vi "LIA Example Host.vi"() -> ()   [LabVIEW 2017]
uses:
  Program Files (x86)/National Instruments/LabVIEW 2017/examples/Lock-In Amplifier/lib/host/Public/pll settings.ctl
  Program Files (x86)/National Instruments/LabVIEW 2017/examples/Lock-In Amplifier/lib/host/Public/lock-in settings.ctl
  Program Files (x86)/National Instruments/LabVIEW 2017/examples/Lock-In Amplifier/lib/interface/Interface FPGA/LIA Host Interface FPGA.lvclass
  C:/Program Files (x86)/National Instruments/LabVIEW 2017/examples/Lock-In Amplifier/lib/interface/Interface/LIA Host Interface.lvclass
  Program Files (x86)/National Instruments/LabVIEW 2017/examples/Lock-In Amplifier/lib/host/Public/fpga type.ctl
  <vilib>/Analysis/4window.llb/windowTd.ctl
  <vilib>/measure/maspectr.llb/Power Spectrum and PSD Export Mode.ctl
  Program Files (x86)/National Instruments/LabVIEW 2017/examples/Lock-In Amplifier/lib/interface/Interface FPGA/Properties/FpgaSession_GET.vi
  <vilib>/Utility/error.llb/Error Cluster From Error Code.vi
  <vilib>/rvi/errors/niLvFpgaAdjustHostInterfaceError.vi
  <vilib>/measure/maspectr.llb/FFT Power Spectrum and PSD for 1 Chan (CDB).vi
  <vilib>/rvi/interface/nirviReadWriteControl/nirviReadWriteControl.xnode
  Program Files (x86)/National Instruments/LabVIEW 2017/examples/Lock-In Amplifier/lib/interface/Interface/LIA Host Interface.lvclass
  Program Files (x86)/National Instruments/LabVIEW 2017/examples/Lock-In Amplifier/lib/host/Lock-In Amplifier Example Host.lvlib
  Program Files (x86)/National Instruments/LabVIEW 2017/examples/Lock-In Amplifier/lib/shared/Lock-In Amplifier Example Shared.lvlib
  NiFpgaLv.dll
  <vilib>/rvi/interface/Simulation/niFpgaSimulationCallBeginRW.vi
  <vilib>/Analysis/NI_AALPro.lvlib
  <vilib>/measure/NI_MAPro.lvlib
  <vilib>/ptbypt/NI_PtbyPt.lvlib
panel:
  in  "Tab Control 2":enum32{"Page 1"}(tab)
  in  "dpll.m 0":i8=-20
  in  "lock-in.decimator 0":enum16{"CIC", "FIR", "None"}(ring)=enum."FIR"
  in  "averaging parameters":T1={"averaging mode"=enum."No averaging", "weighting mode"=enum."Exponential", "number of averages"=10}
  in  "restart averaging (F)":bool
  out "lock-in.max-min":dbl=1.9775797561733533e-07 caption="Deviation" format="%#_6p"
  out "lock-in.min":dbl=1.9775797561733533e-07 caption="Deviation" format="%#_6p"
  out "lock-in.max":dbl=1.9775797561733533e-07 caption="Deviation" format="%#_6p"
  in  "Tab Control 1":enum32{"Page 1", "Page 2"}(tab)
  out "max value":dbl
  out "Waveform Graph 2":cluster{"f0":dbl, "df":dbl, "magnitude":dbl[]}(graph)
  out "stream.request state 0":T2(ring)
  out "pll.vco output 0":fxp<+/-,48,0> format="%#.18g"
  out "lock-in.cic config 0":cluster{"factor":fxp<+,16,16>, "shift":i16}
  out "stream.num samples 0":u64
  out "stream.state 0":T2(ring)
  out "unscaled data":i64[][](array[numeric])
  out "dpll.vco output 0":fxp<+/-,48,0> format="%#.18g"
  out "dpll.config 0":T3
  out "Waveform Graph":cluster{"f0":dbl, "df":dbl, "magnitude":dbl[]}[](graph)
  in  "app.quit":bool
  in  "lock-in.boxcar length 0":u32=2048 caption="Boxar Length"
  in  "app.tab 0":enum32{"Lock-In", "PLL"}(tab)
  in  "lock-in.manual carrier 0":dbl=100000.0 caption="Carrier" format="%_8p"
  in  "lock-in.decimation 0":i32=2048 caption="Decimation"
  in  "lock-in.source 0":enum16{"AI 0", "AI 1", "AI 2", "AI 3"}(ring)=enum."AI 1" caption="Channel"
  in  "lock-in.carrier 0":T4(ring)=enum."DPLL 0" caption="Carrier Source"
  in  "pll.source 0":enum16{"AI 0", "AI 1", "AI 2", "AI 3"}(ring) caption="Source"
  in  "pll.q frequency 0":dbl=100000.0 caption="Q Frequency" format="%#_6p"
  in  "pll.reset 0":bool caption="PLL Reset"
  in  "rio device":tag="PXI1Slot8" caption="Resource"
  in  "lock-in.reset boxar 0":bool
  out "lock-in.deviation 1":dbl=1.9775797561733533e-07 caption="Deviation" format="%#_6p"
  out "lock-in.amplitude 0":dbl=8.221341747482856e-05 caption="Result" format="%#_12p"
  in  "lock-in.boxcar lookback 0":i32=1024 caption="Windows to Average"
  out "Result":cluster{"mean":dbl, "trace":dbl}(graph)={"mean"=8.221341747482856e-05, "trace"=8.36741779633565e-05}
  # "NI Lock-In Amplifier Reference Example"
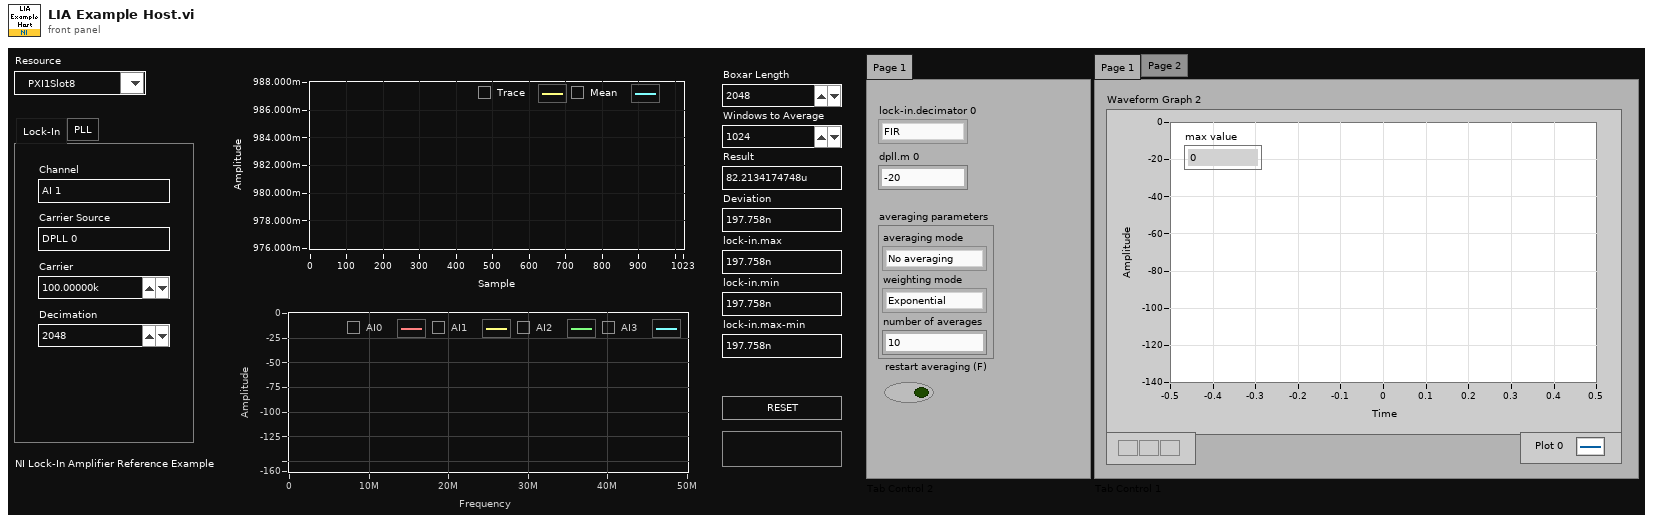
[diagram p1: front panel]
types:
  T1 = cluster{"averaging mode":enum16{"No averaging", "Vector averaging", "RMS averaging", "Peak hold"}, "weighting mode":enum16{"Linear", "Exponential"}, "number of averages":u32}
  T2 = enum8{"Idle", "Finite Transfer", "Continuous", "Done", "Error", "Not Ready", "Cancel"}
  T3 = cluster{"highLevel":fxp<+/-,18,1>, "lowLevel":fxp<+/-,18,1>, "trigger slope":enum8{"Positive", "Negative"}}
  T4 = enum16{"Manual 0", "Manual 1", "Manual 2", "Manual 3", "PLL 0", "PLL 1", "DPLL 0", "DPLL 1"}
  T5 = typedef "Lock-In Amplifier Example Host.lvlib/lock-in settings.ctl" = cluster{"decimation":i32, "source":i32, "carrier source":i32, "carrier":dbl}
  T6 = typedef "Lock-In Amplifier Example Host.lvlib/pll settings.ctl" = cluster{"source":i32, "q frequency":dbl}
  T7 = typedef "Lock-In Amplifier Example Host.lvlib/fpga type.ctl" = refnum<k20>
  T8 = typedef "NI_MAPro.lvlib/Power Spectrum and PSD Export Mode.ctl" = u16
  T9 = typedef "NI_AALPro.lvlib/windowTd.ctl" = u32
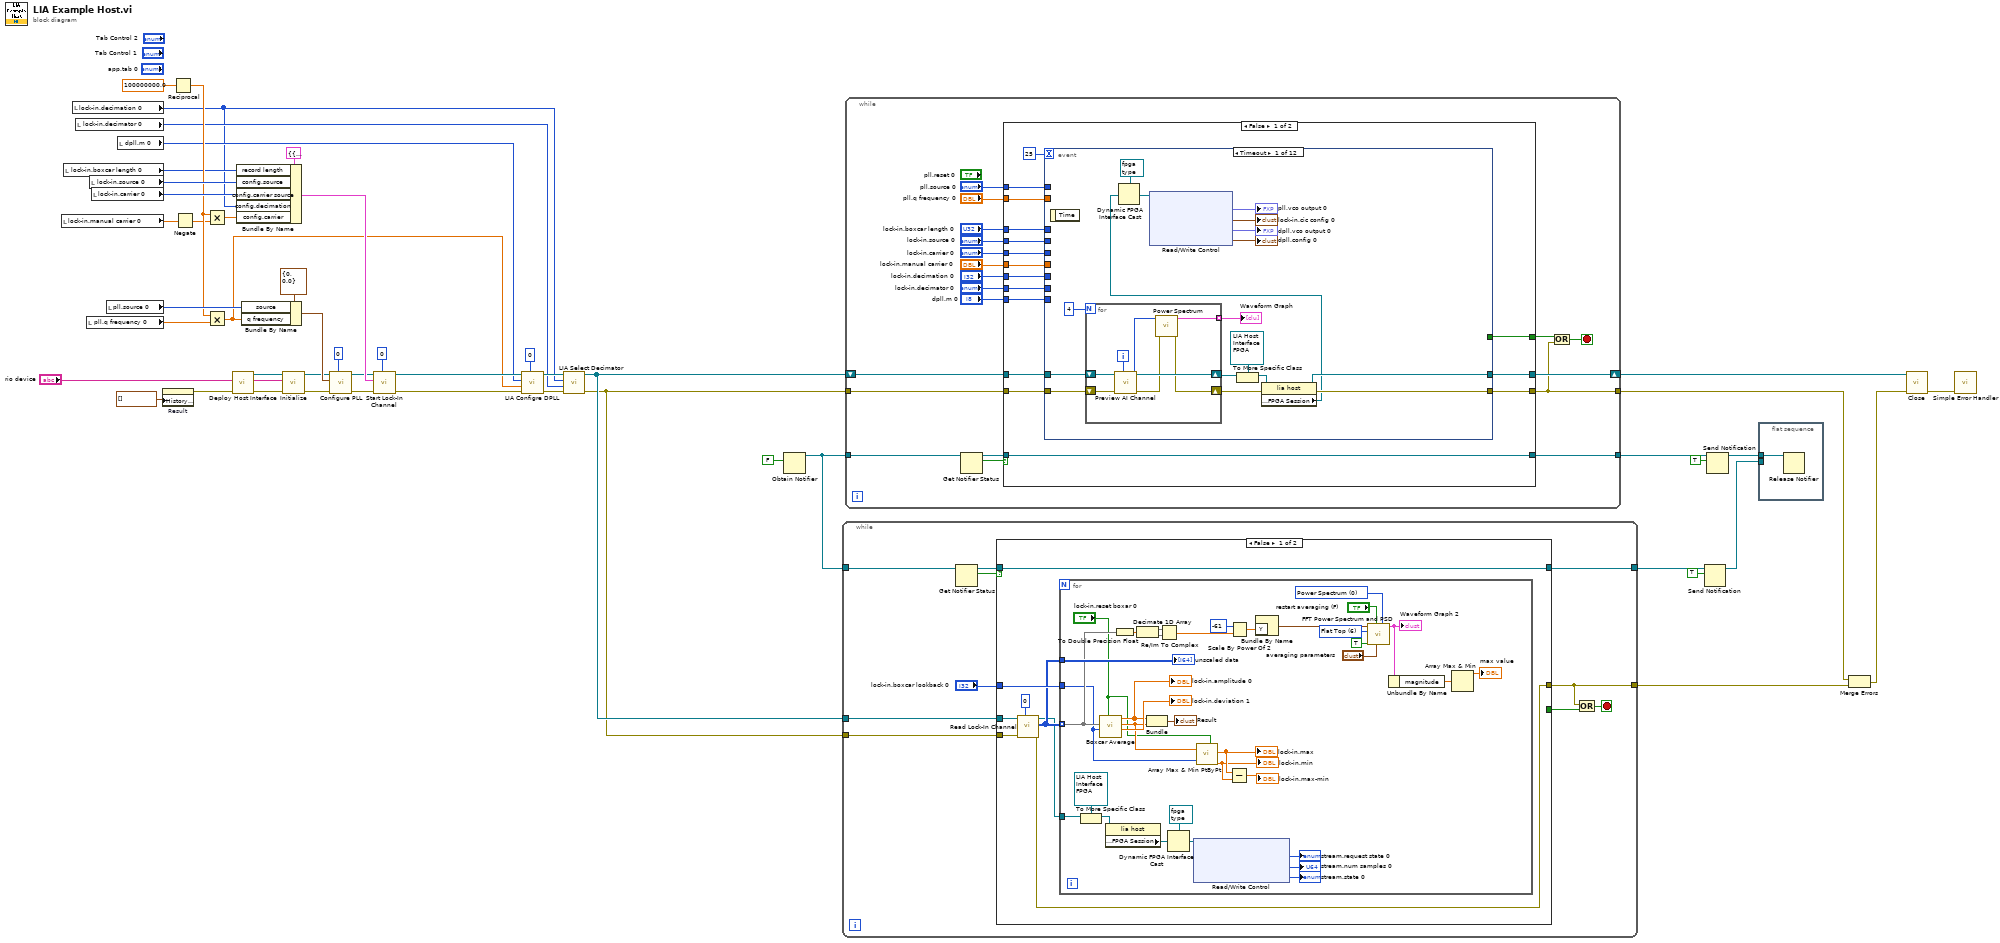
[diagram p0: block diagram]
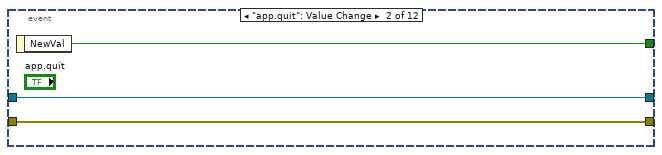
[diagram p2: hidden frame]
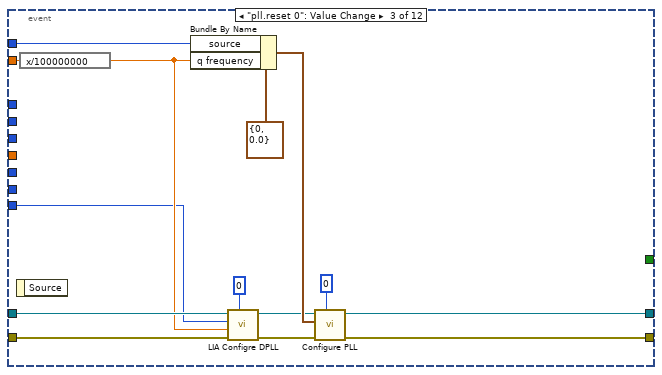
[diagram p3: hidden frame]
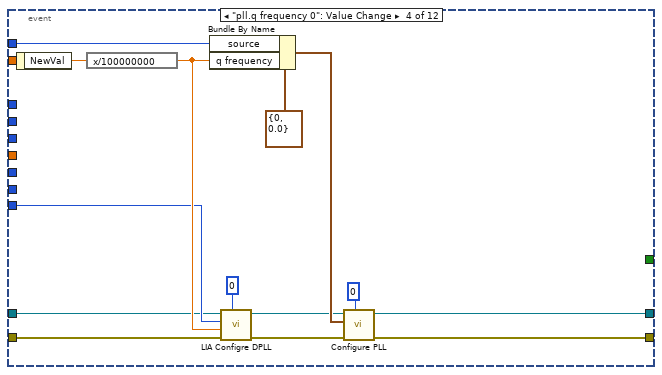
[diagram p4: hidden frame]
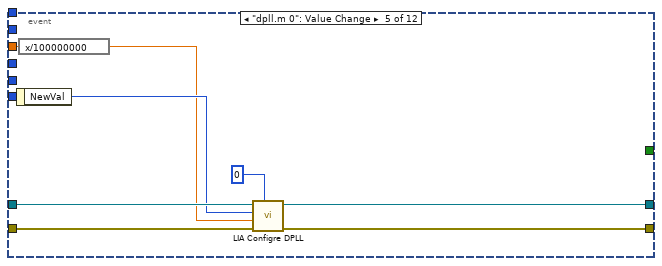
[diagram p5: hidden frame]
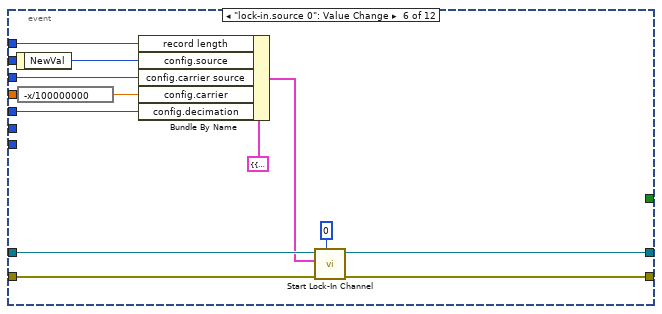
[diagram p6: hidden frame]
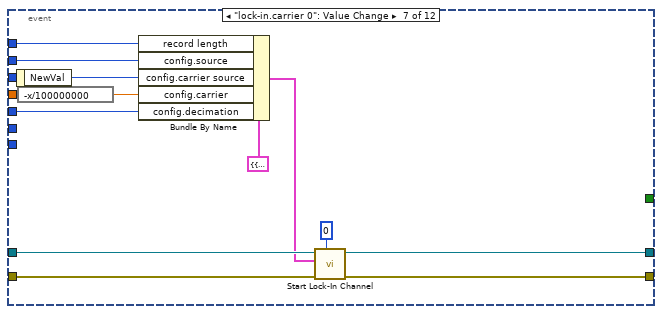
[diagram p7: hidden frame]
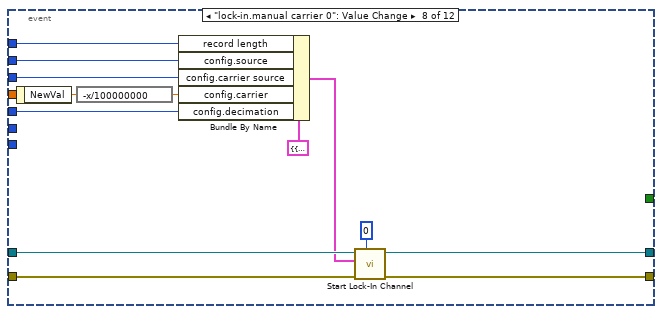
[diagram p8: hidden frame]
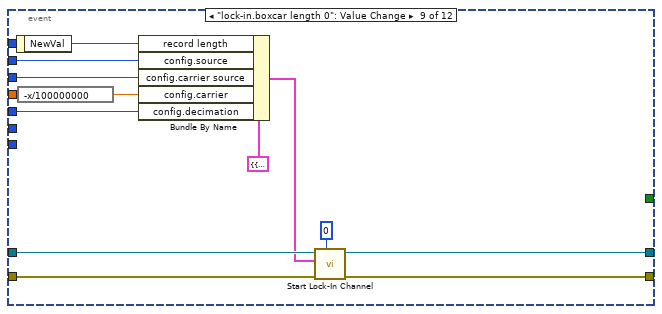
[diagram p9: hidden frame]
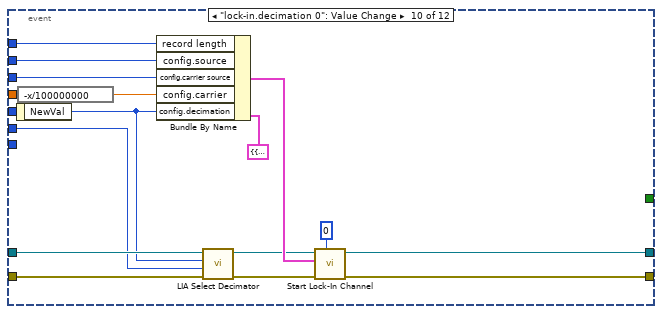
[diagram p10: hidden frame]
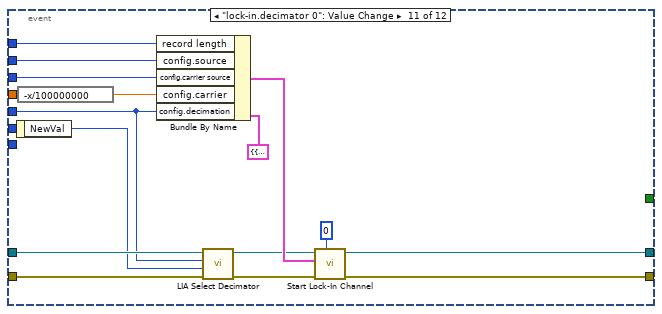
[diagram p11: hidden frame]
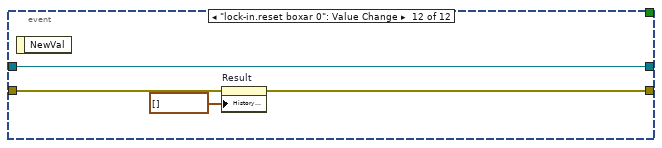
[diagram p12: hidden frame]
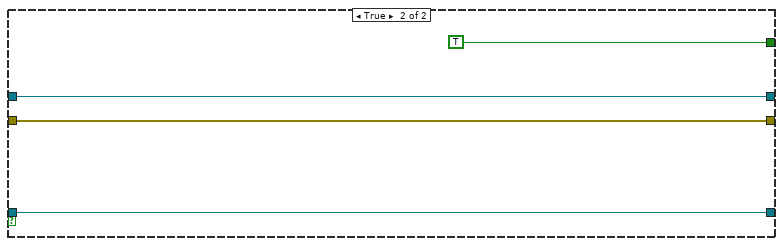
[diagram p13: hidden frame]
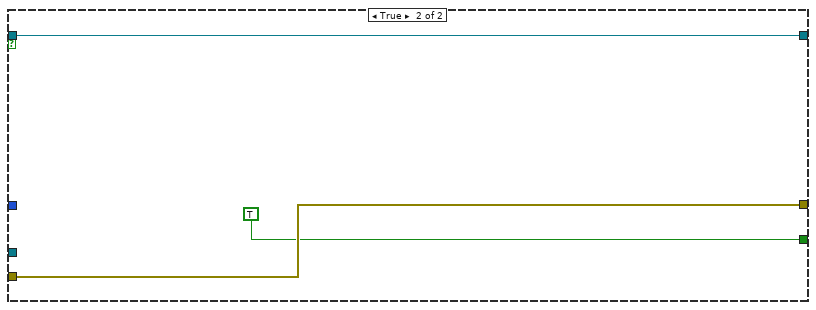
[diagram p14: hidden frame]
diagram:
  n1 = local read "lock-in.manual carrier 0"() -> (w43:dbl)
  n2 = local read "lock-in.boxcar length 0"() -> (w23:u32)
  n3 = local read "lock-in.decimation 0"() -> (w2:i32)
  n4 = local read "lock-in.decimator 0"() -> (w4:enum16{"CIC", "FIR", "None"})
  n5 = local read "pll.q frequency 0"() -> (w46:dbl)
  n6 = local read "lock-in.source 0"() -> (w50:enum16{"AI 0", "AI 1", "AI 2", "AI 3"})
  n7 = local read "lock-in.carrier 0"() -> (w49:T4)
  n8 = local read "pll.source 0"() -> (w47:enum16{"AI 0", "AI 1", "AI 2", "AI 3"})
  n9 = local read "dpll.m 0"() -> (w3:i8)
  n10 = property on="Result" class="WFChart (strict)"("History Data"=cluster{"mean":dbl, "trace":dbl}[] []) -> (error out=w18:errorcluster)  [unwired: 2 in, 1 out]
  n11 = Reciprocal(x=100000000.0) -> (1/x=w44:dbl)
  n12 = Negate(x=w43) -> (-x=w13:dbl)
  n13 = Multiply(x=w44, y=w13) -> (x*y=w11:dbl)
  n14 = Multiply(x=w44, y=w46) -> (x*y=w1:dbl)
  n15 = call "Deploy Host Interface.vi"("error in"=w18, "resource"="rio device") -> ("error out"=w19:errorcluster, "resource out"=w20:string, "lia host interface"=w21:refnum<class "LIA Host Interface.lvclass">)  [unwired: 7 in]
  n16 = Bundle By Name(cluster=cluster{"config":T5, "record length":u32} {"config"={"decimation"=0, "source"=0, "carrier source"=0, "carrier"=0.0}, "record length"=0} ("config"), "record length"=w23, "config.source"=w50, "config.carrier source"=w49, "config.decimation"=w2, "config.carrier"=w11) -> (w24:cluster{"config":T5, "record length":u32})
  n17 = Bundle By Name(cluster=T6 {"source"=0, "q frequency"=0.0} ("config"), "source"=w47, "q frequency"=w1) -> (w42:T6)
  n18 = call-dynamic "Initialize.vi"("error in"=w19, "resource"=w20, "lia host in"=w21) -> ("error out"=w28:errorcluster, "lia host out"=w29:refnum<class "LIA Host Interface.lvclass">)  [unwired: 7 in]
  n19 = call-dynamic "Configure PLL.vi"("instance"=0 ("index"), "error in"=w28, "config"=w42, "lia host in"=w29) -> ("error out"=w16:errorcluster, "lia host out"=w15:refnum<class "LIA Host Interface.lvclass">)  [unwired: 6 in]
  n20 = call-dynamic "Start Lock-In Channel.vi"("instance"=0 ("index"), "error in"=w16, "config"=w24, "lia host in"=w15) -> ("error out"=w12:errorcluster, "lia host out"=w9:refnum<class "LIA Host Interface.lvclass">)  [unwired: 6 in]
  n21 = call "LIA Configre DPLL.vi"("dpll.channel 0"=0, "error in (no error)"=w12, "dpll.q 0"=w1, "dpll.m 0"=w3, "LIA Host Interface in"=w9) -> ("error out"=w6:errorcluster, "LIA Host Interface Out"=w8:refnum<class "LIA Host Interface.lvclass">)  [unwired: 5 in]
  n22 = call "LIA Select Decimator.vi"("error in (no error)"=w6, "lock-in.decimator 0"=w4, "lock-in.decimation 0"=w2, "LIA Host Interface in"=w8) -> ("error out"=w5:errorcluster, "LIA Host Interface out"=w7:refnum<class "LIA Host Interface.lvclass">)  [unwired: 6 in]
  n23 = Obtain Notifier(notification data type=FALSE) -> (notifier out=w39:refnum<notifier>)  [unwired: 3 in, 2 out]
  n24 = while {
    tunnel: w39 -> [w60]
    tunnel: w7 -> [w57]
    tunnel: w5 -> [w56]
    tunnel: [w55] -> w32
    tunnel: [w52] -> w35
    stop <- w54 stop-if-true
    n25 = Get Notifier Status(notifier=w60) -> (notifier out=w58:refnum<notifier>, current notification=w59:bool)  [unwired: 1 in, 3 out]
    n26 = case shown="False" w59 {
      tunnel: [w65 w106] -> w52
      tunnel: w58 -> [w65 w106]
      tunnel: w57 -> [w68 _]
      tunnel: w56 -> [w67 w105]
      tunnel: [w62 w105] -> w55
      tunnel: [_ TRUE] -> w53
      tunnel: "lock-in.boxcar lookback 0" -> [w64 _]
      frame False {
        n27 = call-dynamic "Read Lock-In Channel.vi"("instance"=0 ("index"), "error in"=w67, "lia host in"=w68) -> ("error out"=w62:errorcluster, "unscaled data"=w63:i64[][], "lia host out"=w61:refnum<class "LIA Host Interface.lvclass">)  [unwired: 6 in]
        n28 = for {
          tunnel: w63 -> [w83] mode=indexing
          tunnel: w64 -> [w77]
          tunnel: w63 -> [w100]
          tunnel: w61 -> [w90]
          w72 = T8 0 items=["Power Spectrum", "Power Spectral Density"] ("export mode")
          w99 = T9 6 items=["Rectangle"=0, "Hanning"=1, "Hamming"=2, "Blackman-Harris"=3, "Exact Blackman"=4, "Blackman"=5, "Flat Top"=6, "4 Term B-Harris "=7, "7 Term B-Harris"=8, "Low Sidelobe"=9, "Blackman Nuttall"=11, "Triangle"=30, "Bartlett-Hanning"=31, "Bohman"=32, "Parzen"=33, "Welch"=34, "Kaiser"=60, "Dolph-Chebyshev"=61, "Gaussian"=62] ("window")
          n29 = To More Specific Class(target class=refnum<class "LIA Host Interface FPGA.lvclass"> refnum ("lia host"), reference=w90) -> (specific class reference=w91:refnum<class "LIA Host Interface FPGA.lvclass">)  [unwired: 1 in, 1 out]
          n30 = call "Boxcar Average.vi"("reset"="lock-in.reset boxar 0", "sample length"=w77, "interleaved iq"=w83) -> ("standard deviation"=→"lock-in.deviation 1":dbl, "trace"=w78:dbl, "mean"=w101:dbl)  [unwired: 6 in]
          "lock-in.amplitude 0" <- w101
          n31 = property class="lia host"(reference=w91) -> ("Properties:FPGA Session"=w88:refnum<k20>)  [unwired: 1 in, 2 out]
          n32 = To Double Precision Float(number=w83) -> (double precision float=w94:dbl[])
          n33 = Decimate 1D Array(w94) -> (w96:dbl[], w95:dbl[])
          n34 = Bundle("mean"=w101, "trace"=w78) -> (→"Result":cluster{"mean":dbl, "trace":dbl})  [unwired: 1 in]
          n35 = Re/Im To Complex(1:w95, 2:w96) -> (0:w93:cdb[])
          n36 = Dynamic FPGA Interface Cast(Session In=T7 refnum ("fpga type"), Type=w88) -> (Session Out=w87:T7)
          n37 = xnode "Read/Write Control"("FPGA VI Reference In"=w87) -> ("stream.request state 0"=→"stream.request state 0":T2, "stream.num samples 0"=→"stream.num samples 0":u64, "stream.state 0"=→"stream.state 0":T2)  [unwired: 1 in, 2 out]
          n38 = call <vilib>:"Array Max & Min PtByPt.vi"("input data point"=w78, "sample length"=w77, "initialize"="lock-in.reset boxar 0") -> ("max value"=w75:dbl, "min value"=w74:dbl)  [unwired: 3 out]
          "lock-in.max" <- w75
          "lock-in.min" <- w74
          n39 = Subtract(x=w75, y=w74) -> (x-y=→"lock-in.max-min":dbl)
          n40 = Scale By Power Of 2(n=i16 -61, x=w93) -> (x*2^n=w80:cdb[])
          n41 = Bundle By Name("Y"=w80) -> (w79:waveform(cdb))  [unwired: 1 in]
          n42 = call-poly <vilib>:"FFT Power Spectrum and PSD.vi"("export mode"=w72, "averaging parameters"="averaging parameters", "restart averaging (F)"="restart averaging (F)", "dB On (F)"=TRUE, "window"=w99, "time signal"=w79) -> ("Power Spectrum / PSD"=w70:cluster{"f0":dbl, "df":dbl, "magnitude":dbl[]})  [unwired: 2 in, 3 out]
          "Waveform Graph 2" <- w70
          n43 = Unbundle By Name(w70) -> ("magnitude"=w69:dbl[])
          n44 = Array Max & Min(array=w69) -> (max value=→"max value":dbl)  [unwired: 3 out]
          "unscaled data" <- w100
        }
      }
      frame True {
      }
    }
    n45 = Or(x=w55, y=w53) -> (x .or. y?=w54:bool)
  }
  n46 = while {
    tunnel: w5 -> [w125]
    shift-right: [w116] -> w41
    shift-left: w7 -> [w124]
    tunnel: [w112] -> w31
    tunnel: w39 -> [w115]
    tunnel: [w110] -> w38
    stop <- w123 stop-if-true
    n47 = Get Notifier Status(notifier=w115) -> (notifier out=w114:refnum<notifier>, current notification=w113:bool)  [unwired: 1 in, 3 out]
    n48 = case shown="False" w113 {
      tunnel: w125 -> [w141 w296]
      tunnel: w124 -> [w140 w297]
      tunnel: [w139 w296] -> w112
      tunnel: "lock-in.manual carrier 0" -> [w137 _]
      tunnel: "lock-in.decimation 0" -> [w136 _]
      tunnel: "lock-in.source 0" -> [w135 _]
      tunnel: "lock-in.carrier 0" -> [w134 _]
      tunnel: "pll.source 0" -> [w133 _]
      tunnel: "pll.q frequency 0" -> [w132 _]
      tunnel: [w131 w297] -> w116
      tunnel: w114 -> [w129 w294]
      tunnel: [w130 TRUE] -> w111
      tunnel: [w129 w294] -> w110
      tunnel: "lock-in.boxcar length 0" -> [w128 _]
      tunnel: "lock-in.decimator 0" -> [w127 _]
      tunnel: "dpll.m 0" -> [w126 _]
      frame False {
        n49 = event shown="[0] Timeout" {
          selector: _ -> [_ _ _ _ _ _ _ _ _ _ _ _]
          dyn-events: _ -> [_ _ _ _ _ _ _ _ _ _ _ _]
          timeout: 25 -> [_ _ _ _ _ _ _ _ _ _ _ _]
          tunnel: w141 -> [w157 w168 w173 w184 w200 w214 w228 w241 w253 w262 w278 w293]
          tunnel: w140 -> [w158 w169 w175 w185 w205 w212 w226 w239 w251 w260 w276 w290]
          tunnel: [w149 w168 w183 w193 w198 w213 w227 w240 w252 w270 w286 w292] -> w139
          tunnel: w135 -> [_ _ _ _ _ _ w219 w232 w245 w267 w283 _]
          tunnel: w134 -> [_ _ _ _ _ w217 _ w243 w256 w272 w288 _]
          tunnel: w137 -> [_ _ _ _ w202 w216 w230 _ w255 w271 w287 _]
          tunnel: w136 -> [_ _ _ _ _ w215 w229 w242 w254 _ w274 _]
          tunnel: w133 -> [_ _ w180 w196 _ _ _ _ _ _ _ _]
          tunnel: w132 -> [_ _ w177 _ _ _ _ _ _ _ _ _]
          tunnel: [w150 w169 w178 w194 w199 w211 w225 w238 w250 w269 w285 w290] -> w131
          tunnel: [_ w167 _ _ _ _ _ _ _ _ _ _] -> w130
          tunnel: w128 -> [_ _ _ _ _ w207 w222 w235 _ w265 w281 _]
          tunnel: w127 -> [_ _ _ _ _ _ _ _ _ w258 _ _]
          tunnel: w126 -> [_ _ w170 w188 _ _ _ _ _ _ _ _]
          event Timeout {
            n50 = event-data() -> ()  [unwired: 1 in, 1 out]
            n51 = for {
              N: 4 -> [_]
              shift-right: [w164] -> w152
              shift-left: w158 -> [w166]
              shift-right: [w161] -> w151
              shift-left: w157 -> [w165]
              tunnel: [w159] -> w155 mode=indexing
              i -> [w163]
              n52 = call-dynamic "Preview AI Channel.vi"("instance"=w163, "error in"=w165, "lia host in"=w166) -> ("error out"=w162:errorcluster, "samples"=w160:i16[], "lia host out"=w164:refnum<class "LIA Host Interface.lvclass">)  [unwired: 6 in]
              n53 = call "Power Spectrum.vi"("error in"=w162, "ai data"=w160) -> ("error out"=w161:errorcluster, "magnitude"=w159:cluster{"f0":dbl, "df":dbl, "magnitude":dbl[]})  [unwired: 8 in]
            }
            "Waveform Graph" <- w155
            n54 = To More Specific Class(target class=refnum<class "LIA Host Interface FPGA.lvclass"> refnum ("lia host"), reference=w152) -> (specific class reference=w154:refnum<class "LIA Host Interface FPGA.lvclass">)  [unwired: 1 in, 1 out]
            n55 = property class="lia host"(reference=w154, error in=w151) -> (reference out=w150:refnum<class "LIA Host Interface FPGA.lvclass">, error out=w149:errorcluster, "Properties:FPGA Session"=w148:refnum<k20>)
            n56 = Dynamic FPGA Interface Cast(Session In=T7 refnum ("fpga type"), Type=w148) -> (Session Out=w147:T7)
            n57 = xnode "Read/Write Control"("FPGA VI Reference In"=w147) -> ("pll.vco output 0"=→"pll.vco output 0":fxp<+/-,48,0>, "lock-in.cic config 0"=→"lock-in.cic config 0":cluster{"factor":fxp<+,16,16>, "shift":i16}, "dpll.vco output 0"=→"dpll.vco output 0":fxp<+/-,48,0>, "dpll.config 0"=→"dpll.config 0":T3)  [unwired: 1 in, 2 out]
          }
          event "app.quit": Value Change {
            n58 = event-data() -> ("NewVal"=w167:bool)  [unwired: 1 in]
          }
          event "pll.reset 0": Value Change {
            n59 = event-data() -> ()  [unwired: 1 in, 1 out]
            n60 = expression code="x/100000000"(w177) -> (w171:dbl)
            n61 = Bundle By Name(cluster=T6 {"source"=0, "q frequency"=0.0} ("config"), "source"=w180, "q frequency"=w171) -> (w179:T6)
            n62 = call "LIA Configre DPLL.vi"("dpll.channel 0"=0, "error in (no error)"=w173, "dpll.q 0"=w171, "dpll.m 0"=w170, "LIA Host Interface in"=w175) -> ("error out"=w172:errorcluster, "LIA Host Interface Out"=w174:refnum<class "LIA Host Interface.lvclass">)  [unwired: 5 in]
            n63 = call-dynamic "Configure PLL.vi"("instance"=0 ("index"), "error in"=w172, "config"=w179, "lia host in"=w174) -> ("error out"=w183:errorcluster, "lia host out"=w178:refnum<class "LIA Host Interface.lvclass">)  [unwired: 6 in]
          }
          event "pll.q frequency 0": Value Change {
            n64 = event-data() -> ("NewVal"=w195:dbl)  [unwired: 1 in]
            n65 = expression code="x/100000000"(w195) -> (w189:dbl)
            n66 = Bundle By Name(cluster=T6 {"source"=0, "q frequency"=0.0} ("config"), "source"=w196, "q frequency"=w189) -> (w192:T6)
            n67 = call "LIA Configre DPLL.vi"("dpll.channel 0"=0, "error in (no error)"=w184, "dpll.q 0"=w189, "dpll.m 0"=w188, "LIA Host Interface in"=w185) -> ("error out"=w186:errorcluster, "LIA Host Interface Out"=w187:refnum<class "LIA Host Interface.lvclass">)  [unwired: 5 in]
            n68 = call-dynamic "Configure PLL.vi"("instance"=0, "error in"=w186, "config"=w192, "lia host in"=w187) -> ("error out"=w193:errorcluster, "lia host out"=w194:refnum<class "LIA Host Interface.lvclass">)  [unwired: 6 in]
          }
          event "dpll.m 0": Value Change {
            n69 = event-data() -> ("NewVal"=w203:i8)  [unwired: 1 in]
            n70 = expression code="x/100000000"(w202) -> (w201:dbl)
            n71 = call "LIA Configre DPLL.vi"("dpll.channel 0"=0, "error in (no error)"=w200, "dpll.q 0"=w201, "dpll.m 0"=w203, "LIA Host Interface in"=w205) -> ("error out"=w198:errorcluster, "LIA Host Interface Out"=w199:refnum<class "LIA Host Interface.lvclass">)  [unwired: 5 in]
          }
          event "lock-in.source 0": Value Change {
            n72 = event-data() -> ("NewVal"=w209:enum16{"AI 0", "AI 1", "AI 2", "AI 3"})  [unwired: 1 in]
            n73 = expression code="-x/100000000"(w216) -> (w218:dbl)
            n74 = Bundle By Name(cluster=cluster{"config":T5, "record length":u32} {"config"={"decimation"=0, "source"=0, "carrier source"=0, "carrier"=0.0}, "record length"=0} ("config"), "record length"=w207, "config.source"=w209, "config.carrier source"=w217, "config.carrier"=w218, "config.decimation"=w215) -> (w206:cluster{"config":T5, "record length":u32})
            n75 = call-dynamic "Start Lock-In Channel.vi"("instance"=0 ("index"), "error in"=w214, "config"=w206, "lia host in"=w212) -> ("error out"=w213:errorcluster, "lia host out"=w211:refnum<class "LIA Host Interface.lvclass">)  [unwired: 6 in]
          }
          event "lock-in.carrier 0": Value Change {
            n76 = event-data() -> ("NewVal"=w220:T4)  [unwired: 1 in]
            n77 = expression code="-x/100000000"(w230) -> (w231:dbl)
            n78 = Bundle By Name(cluster=cluster{"config":T5, "record length":u32} {"config"={"decimation"=0, "source"=0, "carrier source"=0, "carrier"=0.0}, "record length"=0} ("config"), "record length"=w222, "config.source"=w219, "config.carrier source"=w220, "config.carrier"=w231, "config.decimation"=w229) -> (w221:cluster{"config":T5, "record length":u32})
            n79 = call-dynamic "Start Lock-In Channel.vi"("instance"=0 ("index"), "error in"=w228, "config"=w221, "lia host in"=w226) -> ("error out"=w227:errorcluster, "lia host out"=w225:refnum<class "LIA Host Interface.lvclass">)  [unwired: 6 in]
          }
          event "lock-in.manual carrier 0": Value Change {
            n80 = event-data() -> ("NewVal"=w233:dbl)  [unwired: 1 in]
            n81 = expression code="-x/100000000"(w233) -> (w244:dbl)
            n82 = Bundle By Name(cluster=cluster{"config":T5, "record length":u32} {"config"={"decimation"=0, "source"=0, "carrier source"=0, "carrier"=0.0}, "record length"=0} ("config"), "record length"=w235, "config.source"=w232, "config.carrier source"=w243, "config.carrier"=w244, "config.decimation"=w242) -> (w234:cluster{"config":T5, "record length":u32})
            n83 = call-dynamic "Start Lock-In Channel.vi"("instance"=0 ("index"), "error in"=w241, "config"=w234, "lia host in"=w239) -> ("error out"=w240:errorcluster, "lia host out"=w238:refnum<class "LIA Host Interface.lvclass">)  [unwired: 6 in]
          }
          event "lock-in.boxcar length 0": Value Change {
            n84 = event-data() -> ("NewVal"=w246:u32)  [unwired: 1 in]
            n85 = expression code="-x/100000000"(w255) -> (w257:dbl)
            n86 = Bundle By Name(cluster=cluster{"config":T5, "record length":u32} {"config"={"decimation"=0, "source"=0, "carrier source"=0, "carrier"=0.0}, "record length"=0} ("config"), "record length"=w246, "config.source"=w245, "config.carrier source"=w256, "config.carrier"=w257, "config.decimation"=w254) -> (w247:cluster{"config":T5, "record length":u32})
            n87 = call-dynamic "Start Lock-In Channel.vi"("instance"=0 ("index"), "error in"=w253, "config"=w247, "lia host in"=w251) -> ("error out"=w252:errorcluster, "lia host out"=w250:refnum<class "LIA Host Interface.lvclass">)  [unwired: 6 in]
          }
          event "lock-in.decimation 0": Value Change {
            n88 = event-data() -> ("NewVal"=w259:i32)  [unwired: 1 in]
            n89 = expression code="-x/100000000"(w271) -> (w273:dbl)
            n90 = Bundle By Name(cluster=cluster{"config":T5, "record length":u32} {"config"={"decimation"=0, "source"=0, "carrier source"=0, "carrier"=0.0}, "record length"=0} ("config"), "record length"=w265, "config.source"=w267, "config.carrier source"=w272, "config.carrier"=w273, "config.decimation"=w259) -> (w264:cluster{"config":T5, "record length":u32})
            n91 = call "LIA Select Decimator.vi"("error in (no error)"=w262, "lock-in.decimator 0"=w258, "lock-in.decimation 0"=w259, "LIA Host Interface in"=w260) -> ("error out"=w261:errorcluster, "LIA Host Interface out"=w263:refnum<class "LIA Host Interface.lvclass">)  [unwired: 6 in]
            n92 = call-dynamic "Start Lock-In Channel.vi"("instance"=0 ("index"), "error in"=w261, "config"=w264, "lia host in"=w263) -> ("error out"=w270:errorcluster, "lia host out"=w269:refnum<class "LIA Host Interface.lvclass">)  [unwired: 6 in]
          }
          event "lock-in.decimator 0": Value Change {
            n93 = event-data() -> ("NewVal"=w275:enum16{"CIC", "FIR", "None"})  [unwired: 1 in]
            n94 = expression code="-x/100000000"(w287) -> (w289:dbl)
            n95 = Bundle By Name(cluster=cluster{"config":T5, "record length":u32} {"config"={"decimation"=0, "source"=0, "carrier source"=0, "carrier"=0.0}, "record length"=0} ("config"), "record length"=w281, "config.source"=w283, "config.carrier source"=w288, "config.carrier"=w289, "config.decimation"=w274) -> (w280:cluster{"config":T5, "record length":u32})
            n96 = call "LIA Select Decimator.vi"("error in (no error)"=w278, "lock-in.decimator 0"=w275, "lock-in.decimation 0"=w274, "LIA Host Interface in"=w276) -> ("error out"=w277:errorcluster, "LIA Host Interface out"=w279:refnum<class "LIA Host Interface.lvclass">)  [unwired: 6 in]
            n97 = call-dynamic "Start Lock-In Channel.vi"("instance"=0 ("index"), "error in"=w277, "config"=w280, "lia host in"=w279) -> ("error out"=w286:errorcluster, "lia host out"=w285:refnum<class "LIA Host Interface.lvclass">)  [unwired: 6 in]
          }
          event "lock-in.reset boxar 0": Value Change {
            n98 = event-data() -> ()  [unwired: 1 in, 1 out]
            n99 = property on="Result" class="WFChart (strict)"(error in=w293, "History Data"=cluster{"mean":dbl, "trace":dbl}[] []) -> (error out=w292:errorcluster)  [unwired: 1 in, 1 out]
          }
        }
      }
      frame True {
      }
    }
    n100 = Or(x=w111, y=w112) -> (x .or. y?=w123:bool)
  }
  n101 = Send Notification(notification=TRUE, notifier=w35) -> (notifier out=w33:refnum<notifier>)  [unwired: 1 in, 1 out]
  n102 = Send Notification(notification=TRUE, notifier=w38) -> (notifier out=w34:refnum<notifier>)  [unwired: 1 in, 1 out]
  n103 = flat-sequence {
    tunnel: w34 -> [w298]
    tunnel: w33 -> [_]
    frame #0 {
      n104 = Release Notifier(notifier=w298) -> ()  [unwired: 2 in, 3 out]
    }
  }
  n105 = Merge Errors(w31, w32) -> (w30:errorcluster)
  n106 = call-dynamic "Close.vi"("error in"=w30, "lia host in"=w41) -> ("error out"=w14:errorcluster)  [unwired: 8 in, 1 out]
  n107 = call <vilib>:"Simple Error Handler.vi"("error in (no error)"=w14) -> ()  [unwired: 4 in, 5 out]
